vi "VoltageSourceTree.vi"   [LabVIEW 2019]
uses:
  lvsrc/Instrument Types/VSource/Instrument.VSource.lvclass
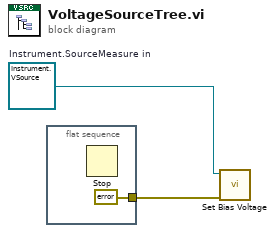
[diagram p0: block diagram]
diagram:
  w1 = refnum<class "Instrument.VSource.lvclass"> refnum  # Instrument.SourceMeasure in
  n1 = flat-sequence {
    tunnel: [errorcluster {"status"=FALSE, "code"=0, "source"=""} ("error in (no error)")] -> w2
    frame #0 {
      n2 = Stop() -> ()  [unwired: 1 in]
    }
  }
  n3 = call-dynamic "Set Bias Voltage.vi"("error in (no error)"=w2, "Instrument.VSource in"=w1) -> ()  [unwired: 8 in, 2 out]
